vi "turn unt current.vi"(8 "error in (no error)":errorcluster, 11 "I2C Ref in":T1) -> (0 "error out":errorcluster, 3 "I2C Ref Out":T1, 5 "angle Z":ext)   [LabVIEW 2017]
uses:
  <vilib>/myRIO/Instrument Drivers/Onboard IO/I2C/typedefs/I2C Reference.ctl
  <vilib>/myRIO/Common/Instrument Driver Framework/Utilities/typedefs/myRIO Generic Hardware Reference.ctl
  <vilib>/myRIO/Common/Instrument Driver Framework/Utilities/typedefs/Hardware Version Enum.ctl
  <vilib>/myRIO/Common/Instrument Driver Framework/Utilities/typedefs/myRIO v1.0 Reference.ctl
  <vilib>/myRIO/Common/Instrument Driver Framework/Utilities/typedefs/Generic FPGA Reference.ctl
  <vilib>/myRIO/Common/Instrument Driver Framework/myRIO v1.0/I2C/typedefs/I2C Channels Enum.ctl
  <vilib>/myRIO/Instrument Drivers/Onboard IO/I2C/typedefs/I2C Configuration.ctl
  <vilib>/myRIO/Instrument Drivers/Onboard IO/I2C/typedefs/I2C Transfer Rate.ctl
  <vilib>/myRIO/Instrument Drivers/Onboard IO/I2C/I2C.lvlib
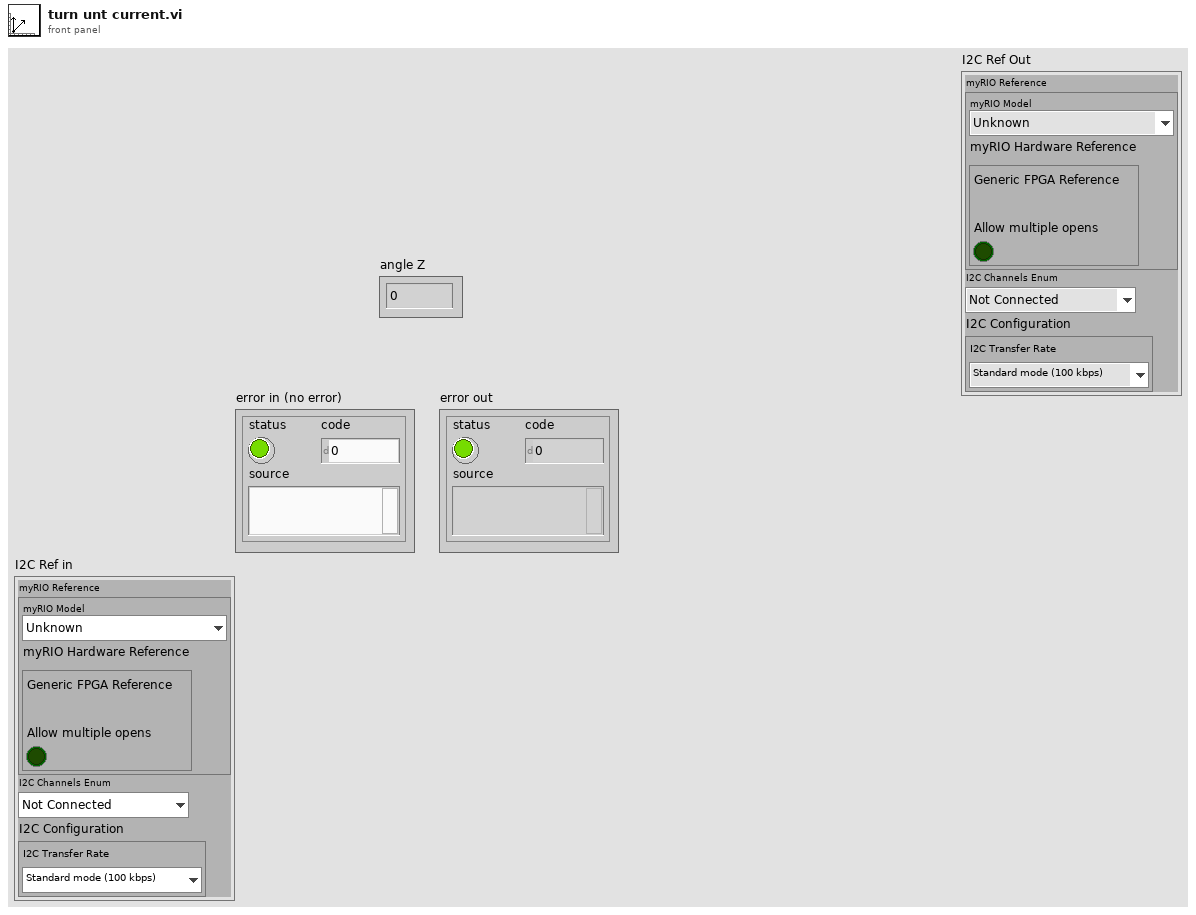
[diagram p1: front panel]
types:
  T1 = typedef "I2C.lvlib/I2C Reference.ctl" = cluster{"myRIO Reference":T2, "I2C Channels Enum":T6, "I2C Configuration":T7}
  T2 = typedef "myRIO Generic Hardware Reference.ctl" = cluster{"myRIO Model":T3, "myRIO Hardware Reference":T4}
  T3 = typedef "Hardware Version Enum.ctl" = enum16{"Unknown", "myRIO-1900", "myRIO-1950", "roboRIO", "NI ELVIS RIO CM"}
  T4 = typedef "myRIO v1.0 Reference.ctl" = cluster{"Generic FPGA Reference":T5, "Allow multiple opens":bool}
  T5 = typedef "Generic FPGA Reference.ctl" = refnum<k20>
  T6 = typedef "I2C Channels Enum.ctl" = enum16{"Not Connected", "A/I2C", "B/I2C", "I2C/I2C"}
  T7 = typedef "I2C.lvlib/I2C Configuration.ctl" = cluster{"I2C Transfer Rate":T8}
  T8 = typedef "I2C.lvlib/I2C Transfer Rate.ctl" = enum16{"Standard mode (100 kbps)", "Fast mode (400 kbps)"}
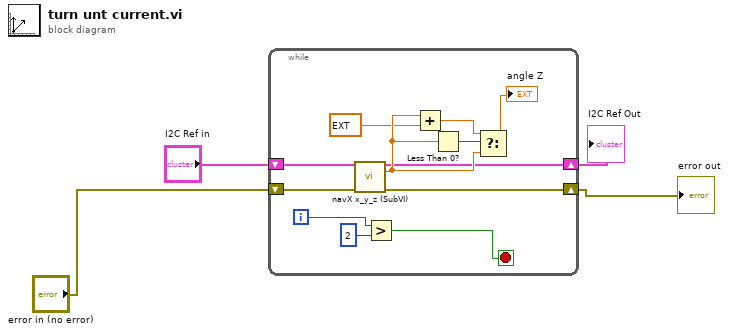
[diagram p0: block diagram]
diagram:
  n1 = while {
    shift-right: [w16] -> w3
    shift-left: "error in (no error)" -> [w14]
    shift-right: [w8] -> w1
    shift-left: "I2C Ref in" -> [w15]
    i -> [w6]
    stop <- w13 stop-if-true
    n2 = call "navX x_y_z (SubVI).vi"("I2C Ref Out in"=w15, "error in (no error)"=w14) -> ("I2C Ref Out out"=w8:T1, "value Z"=w10:ext, "error out"=w16:errorcluster)  [unwired: 9 in, 2 out]
    n3 = Greater?(x=w6, y=2) -> (0:w13:bool)
    n4 = Add(x=w10, y=ext 360.0) -> (x+y=w11:ext)
    n5 = Less Than 0?(x=w10) -> (x < 0?=w12:bool)
    n6 = Select(t=w11, s=w12, f=w10) -> (s? t:f=→"angle Z":ext)
  }
  "error out" <- w3
  "I2C Ref Out" <- w1
